vi "camara y daq.vi"() -> ()   [LabVIEW 2010]
uses:
  <vilib>/sound2/lvsound2.llb/Sound Data Format.ctl
  <vilib>/addons/PixeLINK/Low Level Functions/CAMERA_FEATURES.llb/TDPU-CameraFeatures-PixelFormat.ctl
  <vilib>/vision/Image Controls.llb/IMAQ Image.ctl
  <vilib>/sound2/lvsound2.llb/Sound Output Task ID.ctl
panel:
  in  "seconds to wait":dbl
  out "Image 2":T1
  out "Array":T1[](array[plugin-control])
  in  "Tab Control":enum32{"DAQ", "Sound", "Camara"}(tab)
  out "Waveform DAQ":waveform(dbl)(graph)
  in  "Calibracion DAQ":T2
  in  "DAQ Controls":T3={"Minimum Value"=-10.0, "Maximum Value"=10.0, "Physical Channel"="Dev1/ao0", "DAQ Fs (S/s)"=10000.0} {"Minimum Value" min=-10.0 max=0.0; "Maximum Value" min=0.0 max=10.0}
  in  "tiempo (ms)":dbl
  in  "DAQ?":bool
  in  "Sound Controls":T5={"device ID"=0, "sound format"={"sample rate (S/s)"=44000.0, "number of channels"=2, "bits per sample"=16}, "time (ms)"=200.0}
  in  "Sound?":bool
  in  "Frecuencia":dbl
  out "Waveform Sound":waveform(dbl)(graph)
  in  "Selector":u16(ring) items=["776002034"]
  in  "Streeam?":bool
  out "Camara Funciona?":bool
  out "Contraste":dbl
  out "Image":T1(plugin-control)
  in  "Camara Parameters":T7 {"Pixel Format" items=["PIXEL_FORMAT_MONO8", "PIXEL_FORMAT_MONO16", "PIXEL_FORMAT_YUV422", "PIXEL_FORMAT_BAYER8_GRBG", "PIXEL_FORMAT_BAYER16_GRBG", "PIXEL_FORMAT_RGB24", "PIXEL_FORMAT_RGB48", "PIXEL_FORMAT_BAYER8_RGGB", "PIXEL_FORMAT_BAYER8_GBRG ", "PIXEL_FORMAT_BAYER8_BGGR ", "PIXEL_FORMAT_BAYER16_RGGB ", "PIXEL_FORMAT_BAYER16_GBRG", "PIXEL_FORMAT_BAYER16_BGGR", "PIXEL_FORMAT_RGB32"]}
  in  "stop":bool
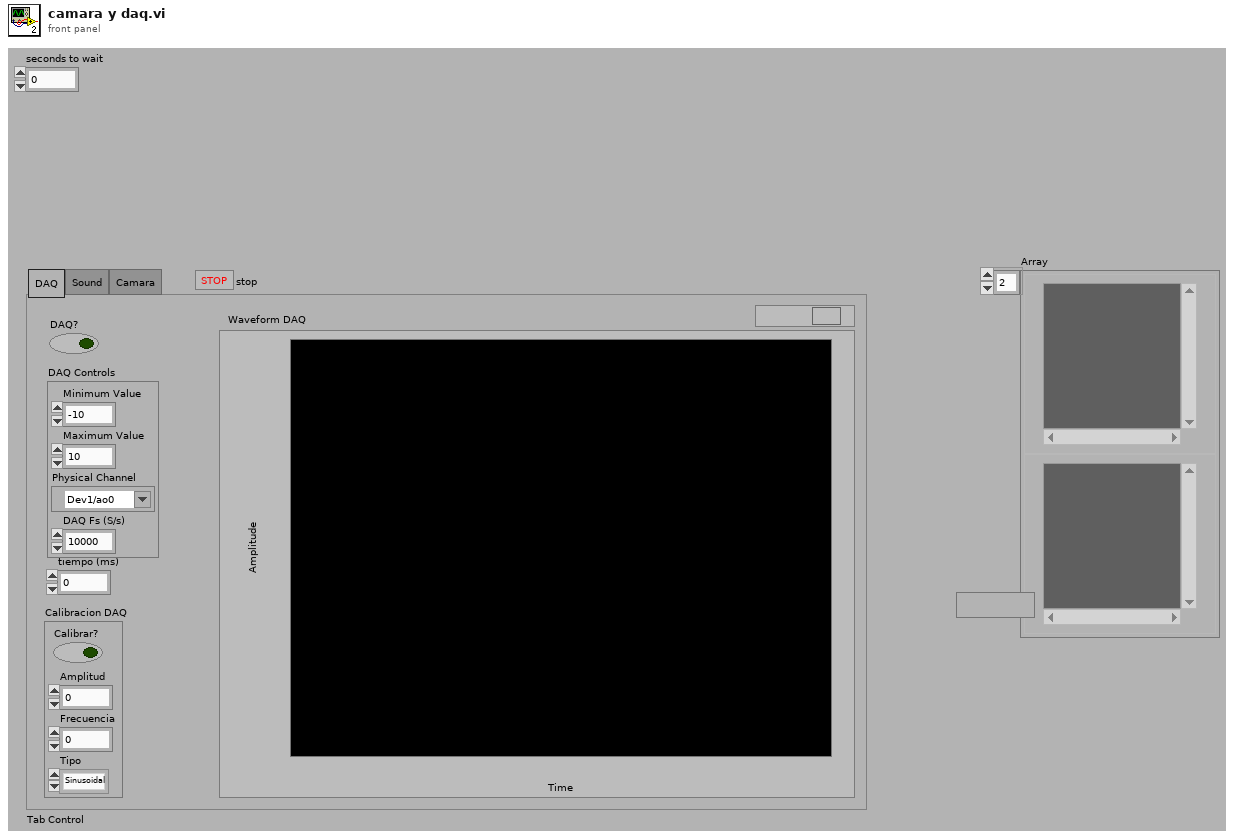
[diagram p1: front panel]
types:
  T1 = typedef "IMAQ Image.ctl" = refnum<image>
  T2 = cluster{"Calibrar?":bool, "Amplitud":dbl, "Frecuencia":dbl, "Tipo":enum16{"Sinusoidal", "Triangular", "Cuadrada"}}
  T3 = cluster{"Minimum Value":dbl, "Maximum Value":dbl, "Physical Channel":tag, "DAQ Fs (S/s)":dbl}
  T4 = typedef "Sound Data Format.ctl" = cluster{"sample rate (S/s)":dbl, "number of channels":i32, "bits per sample":i32}
  T5 = cluster{"device ID":u32, "sound format":T4, "time (ms)":dbl}
  T6 = typedef "TDPU-CameraFeatures-PixelFormat.ctl" = u16
  T7 = cluster{"Exposure Time (ms)":dbl, "Gain (dB)":dbl, "Saturation (%)":dbl, "Sharpness (%)":dbl, "Color Temperature":dbl, "ROI":cluster{"Top":i32, "Left":i32, "Width":i32, "Height":i32}, "White Balance Gain (dB)":cluster{"Red":dbl, "Green":dbl, "Blue":dbl}, "Gamma":dbl, "Pixel Format":T6, "FPS (frames/s)":i32}
  T8 = cluster{"hCamera":u32, "Error":errorcluster, "uSerialNumber OUT":u32}
  T9 = typedef "Sound Output Task ID.ctl" = u32
  T10 = cluster{"task ID":T9, "error":errorcluster, "sound format":T4}
  T11 = cluster{"DAQ Fs (S/s)":dbl, "task":refnum<k21>, "error":errorcluster, "Min Value":dbl, "Max Value":dbl}
  T12 = cluster{"DAQ Limits":cluster{"max":dbl, "min":dbl}, "Control Limits":cluster{"max":dbl, "min":dbl}}
  T13 = cluster{"hCamera":u32, "Error":errorcluster, "uSerialNumber":u32}
  T14 = typedef "Image Type" = u32
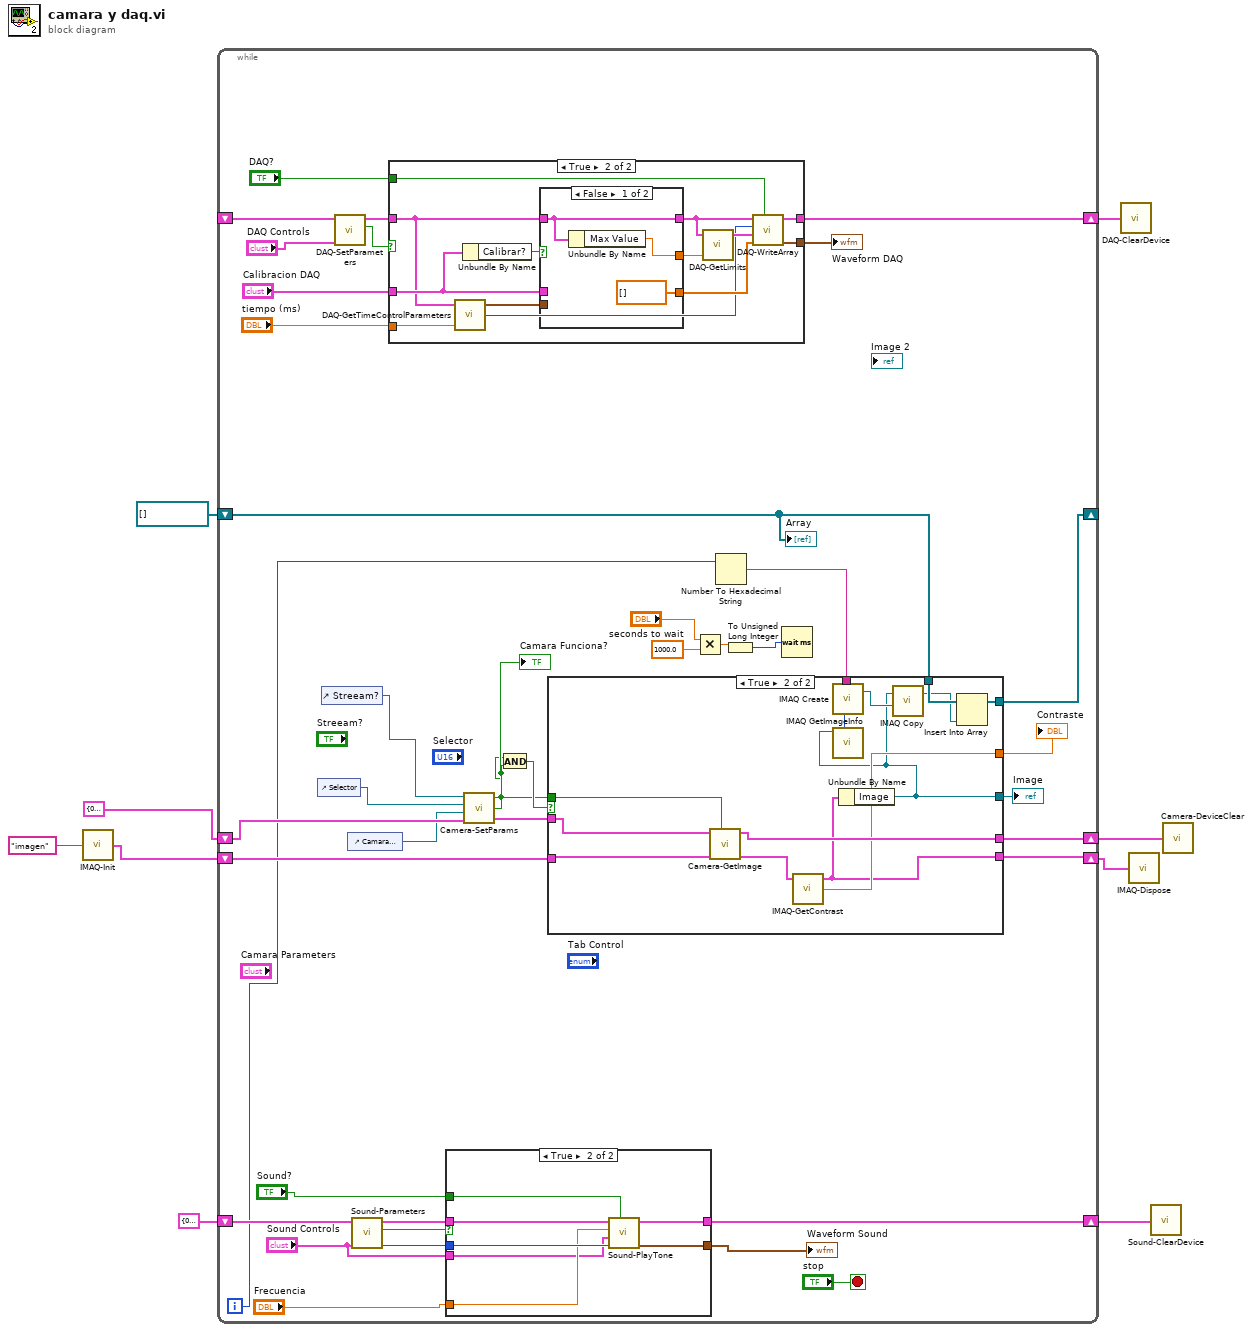
[diagram p0: block diagram]
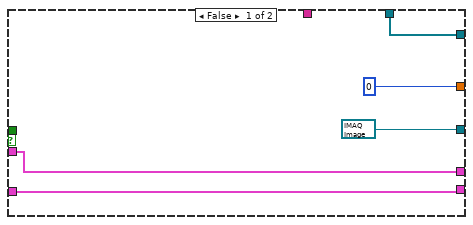
[diagram p2: hidden frame]
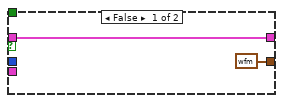
[diagram p3: hidden frame]
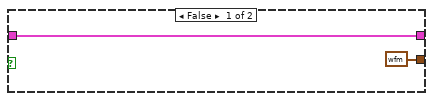
[diagram p4: hidden frame]
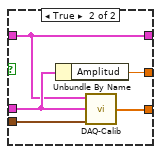
[diagram p5: hidden frame]
diagram:
  n1 = call "IMAQ-Init.vi"("Image Name"="imagen") -> ("Image Device OUT"=w5:cluster{"Image":T1, "errorImage":errorcluster})  [unwired: 2 in, 2 out]
  n2 = while {
    shift-right: [w41] -> w7
    shift-left: _ -> [w42]
    shift-right: [w37] -> w8
    shift-left: T10 {"task ID"=0, "error"={"status"=TRUE, "code"=0, "source"=""}, "sound format"={"sample rate (S/s)"=0.0, "number of channels"=0, "bits per sample"=0}} ("Sound Device OUT") -> [w36]
    shift-right: [w24] -> w2
    shift-left: w5 -> [w27]
    shift-right: [w26] -> w3
    shift-left: T8 {"hCamera"=0, "Error"={"status"=FALSE, "code"=0, "source"=""}, "uSerialNumber OUT"=0} ("Camera Device  IN") -> [w25]
    shift-right: [w10] -> _
    shift-left: T1[] [] -> [w11]
    i -> [w14]
    stop <- "stop" stop-if-true
    n3 = control-ref of="Selector"() -> (w30:refnum<vi>)
    n4 = control-ref of="Streeam?"() -> (w29:refnum<vi>)
    n5 = call "DAQ-SetParameters.vi"("DAQ Controls"="DAQ Controls", "DAQ Device IN"=w42) -> ("En Funcionamiento?"=w35:bool, "DAQ Device OUT"=w47:T11)  [unwired: 4 in]
    n6 = control-ref of="Camara Parameters"() -> (w19:refnum<vi>)
    n7 = call "Sound-Parameters.vi"("Sound Controls"="Sound Controls", "Sound Device IN"=w36) -> ("#samples"=w38:u32, "En funcionamiento?"=w34:bool, "Sound Device OUT"=w39:T10)  [unwired: 3 in]
    n8 = case shown="True" w35 {
      tunnel: "DAQ?" -> [_ w90]
      tunnel: w47 -> [w79 w81]
      tunnel: [waveform(dbl) {"t0"=timestamp(0 s since 1904-01-01), "dt"=1.0, "Y"=[]} ("Waveform Graph") w87] -> w46
      tunnel: "Calibracion DAQ" -> [_ w83]
      tunnel: "tiempo (ms)" -> [_ w85]
      tunnel: [w79 w84] -> w41
      frame False {
      }
      frame True {
        n9 = call "DAQ-GetTimeControlParameters.vi"("tiempo (ms)"=w85, "DAQ Device IN"=w81) -> ("#samples"=w88:u32, "Time Control Parameters"=w89:cluster{"# samples":u32, "tiempos (ms)":dbl})  [unwired: 2 in]
        n10 = Unbundle By Name(w83) -> ("Calibrar?"=w82:bool)
        n11 = case shown="False" w82 {
          tunnel: [dbl[] [] ("Calibration OUT") w100] -> w92
          tunnel: w89 -> [_ w99]
          tunnel: w81 -> [w93 w96]
          tunnel: w83 -> [_ w98]
          tunnel: [w94 w97] -> w86
          tunnel: [w93 w96] -> w80
          frame False {
            n12 = Unbundle By Name(w93) -> ("Max Value"=w94:dbl)
          }
          frame True {
            n13 = Unbundle By Name(w98) -> ("Amplitud"=w97:dbl)
            n14 = call "DAQ-Calib.vi"("Time Control Parameters"=w99, "Calibracion DAQ"=w98, "DAQ Device IN"=w96) -> ("Calibration OUT"=w100:dbl[])  [unwired: 1 in]
          }
        }
        n15 = call "DAQ-GetLimits.vi"("Amplitud"=w86, "DAQ Device IN"=w80) -> ("Limites"=w91:T12)  [unwired: 3 in]
        n16 = call "DAQ-WriteArray.vi"("DAQ?"=w90, "Control Array"=w92, "Limites"=w91, "#samples"=w88, "DAQ Device IN"=w80) -> ("Waveform Graph"=w87:waveform(dbl), "DAQ Device OUT"=w84:T11)  [unwired: 2 in]
      }
    }
    "Waveform DAQ" <- w46
    n17 = case shown="True" w34 {
      tunnel: [waveform(dbl) {"t0"=timestamp(0 s since 1904-01-01), "dt"=1.0, "Y"=[]} ("Waveform") w77] -> w40
      tunnel: w39 -> [w70 w76]
      tunnel: w38 -> [_ w75]
      tunnel: [w70 w74] -> w37
      tunnel: "Sound?" -> [_ w73]
      tunnel: "Frecuencia" -> [_ w72]
      tunnel: "Sound Controls" -> [_ w71]
      frame False {
      }
      frame True {
        n18 = call "Sound-PlayTone.vi"("sound?"=w73, "# samples"=w75, "Sound Controls"=w71, "Frecuencia"=w72, "Sound Device IN"=w76) -> ("Waveform"=w77:waveform(dbl), "Sound Device OUT"=w74:T10)  [unwired: 3 in]
      }
    }
    "Waveform Sound" <- w40
    n19 = call "Camera-SetParams.vi"("Camera Device  IN"=w25, "Camera Parameters"=w19, "Selector"=w30, "Stream?"=w29) -> ("Camera Device OUT"=w28:T13, "Funciona?"=w22:bool, "Stream? OUT"=w21:bool)
    "Camara Funciona?" <- w22
    n20 = And(x=w21, y=w22) -> (x .and. y?=w23:bool)
    n21 = Multiply(x="seconds to wait", y=1000.0) -> (x*y=w16:dbl)
    n22 = Number To Hexadecimal String(2:w14) -> (0:w12:string)  [unwired: 1 in]
    n23 = case shown="True" w23 {
      tunnel: w28 -> [w54 w67]
      tunnel: w21 -> [_ w68]
      tunnel: w27 -> [w53 w66]
      tunnel: [w54 w65] -> w26
      tunnel: [T1 refnum ("Image") w58] -> w13
      tunnel: [w53 w62] -> w24
      tunnel: [u32 0 ("Numeric") w64] -> w20
      tunnel: w12 -> [_ w61]
      tunnel: w11 -> [w50 w57]
      tunnel: [w50 w55] -> w10
      frame False {
      }
      frame True {
        n24 = call "Camera-GetImage.vi"("Streeam"=w68, "Image Device IN"=w66, "Camera Device IN"=w67) -> ("Image Device OUT"=w63:cluster{"Image":T1, "errorImage":errorcluster}, "Camera Device OUT"=w65:T13)  [unwired: 4 in]
        n25 = call "IMAQ-GetContrast.vi"("Image Device IN"=w63) -> ("RMS Contraste"=w64:dbl, "Image Device OUT"=w62:cluster{"Image":T1, "errorImage":errorcluster})  [unwired: 3 in]
        n26 = Unbundle By Name(w62) -> ("Image"=w58:T1)
        n27 = call "IMAQ GetImageInfo"("Image"=w58) -> ("Image Type"=w60:T14)  [unwired: 3 in, 7 out]
        n28 = call "IMAQ Create"("Image Name"=w61, "Image Type"=w60) -> ("New Image"=w59:T1)  [unwired: 3 in, 1 out]
        n29 = call "IMAQ Copy"("Image Dst"=w59, "Image Src"=w58) -> ("Image Dst Out"=w56:T1)  [unwired: 4 in, 1 out]
        n30 = Insert Into Array(array=w57, new element=w56) -> (w55:T1[])  [unwired: 1 in]
      }
    }
    "Image" <- w13
    "Contraste" <- w20
    n31 = To Unsigned Long Integer(number=w16) -> (unsigned 32bit integer=w15:u32)
    n32 = Wait (ms)(milliseconds to wait=w15) -> ()  [unwired: 1 out]
    "Array" <- w11
  }
  n33 = call "DAQ-ClearDevice.vi"("DAQ Device IN"=w7) -> ()
  n34 = call "IMAQ-Dispose.vi"("Image Device IN"=w2) -> ()
  n35 = call "Sound-ClearDevice.vi"("Sound Device OUT"=w8) -> ()
  n36 = call "Camera-DeviceClear.vi"("Camera Device OUT"=w3) -> ()
